vi "getvnames.vi"(2 "Object":u16, 3 "connection reference in":T1) -> (0 "StringsAndValues[]":cluster{"String":string, "Value":u16}[](array[cluster]), 1 "connection reference out":T1)   [LabVIEW 2010]
uses:
  <vilib>/addons/database/Connection.llb/Conn ObjectReference.ctl
  <vilib>/addons/database/NI_Database_API.lvlib
panel:
  in  "error in (no error)":errorcluster
  out "error out":errorcluster
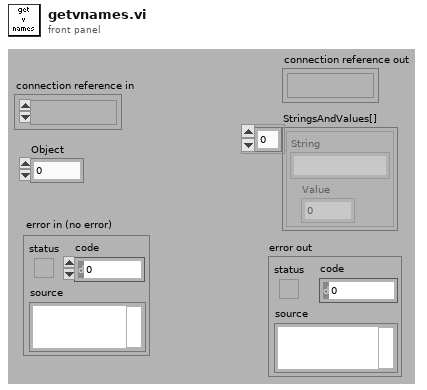
[diagram p1: front panel]
types:
  T1 = typedef "NI_Database_API.lvlib/Conn ObjectReference.ctl" = refnum<k1>
  T2 = cluster{"String":string, "String 2":string, "Value":u16}
  T3 = cluster{"data[0]":variant, "data[1]":variant, "data[2]":variant}
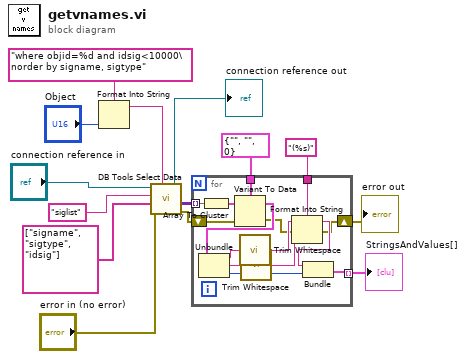
[diagram p0: block diagram]
diagram:
  n1 = Format Into String(format string="where objid=%d and idsig<10000\norder by signame, sigtype" ("initial string"), "Object") -> (resulting string=w7:string)  [unwired: 2 in, 1 out]
  n2 = call <vilib>:"DB Tools Select Data.vi"("condition"=w7, "error in (no error)"="error in (no error)", "columns"=string[] ["signame", "sigtype", "idsig"], "table"="siglist", "connection reference"="connection reference in") -> ("error out"=w3:errorcluster, "data"=w9:variant[][], "connection reference out"=→"connection reference out":T1)  [unwired: 1 in]
  n3 = for {
    tunnel: w9 -> [w29] mode=indexing
    tunnel: T2 {"String"="", "String 2"="", "Value"=0} -> [w27]
    tunnel: "(%s)" ("format string") -> [w23]
    tunnel: [w20] -> w13 mode=indexing
    shift-right: [w15] -> w2
    shift-left: w3 -> [w17]
    n4 = Array To Cluster(array=w29) -> (cluster=w28:T3)
    n5 = Variant To Data(error in=w17, Variant=w28, type=w27) -> (error out=w16:errorcluster, data=w26:T2)
    n6 = Unbundle(w26) -> ("String"=w25:string, "String 2"=w24:string, "Value"=w21:u16)
    n7 = call <vilib>:"Trim Whitespace.vi"("string"=w25) -> ("trimmed string"=w19:string)  [unwired: 1 in]
    n8 = call <vilib>:"Trim Whitespace.vi"("string"=w24) -> ("trimmed string"=w18:string)  [unwired: 1 in]
    n9 = Format Into String(format string=w23, initial string=w19, error in=w16, w18) -> (resulting string=w22:string, error out=w15:errorcluster)
    n10 = Bundle(w22, "Value"=w21) -> (w20:cluster{string, "Value":u16})  [unwired: 1 in]
  }
  "StringsAndValues[]" <- w13
  "error out" <- w2
